vi "Retrieve Unit from Data Report.vi"(8 "error in (no error)":errorcluster, 10 "Row":u16, 11 "report in":refnum<class "NI_report.lvclass">) -> (0 "error out":errorcluster, 2 "data":string, 3 "report out":refnum<class "NI_report.lvclass">)   [LabVIEW 2019]
doc: "For use with Tektronix Excel Data Reports\n\nReturns the text in the Units column for the given Row (Zero Indexed)"
uses:
  <vilib>/Utility/NIReport.llb/NI_report.lvclass
  <vilib>/addons/_office/excel.llb/Excel Get Data (str).vi
  <vilib>/addons/_office/NI_ReportGenerationToolkit.lvlib
  <vilib>/Utility/NIReport.llb/Excel/NI_Excel.lvclass
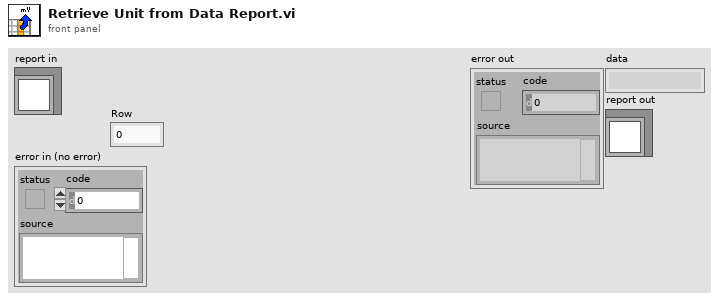
[diagram p1: front panel]
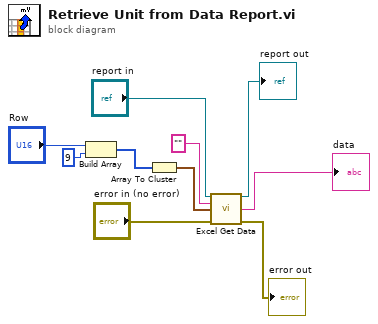
[diagram p0: block diagram]
diagram:
  n1 = Build Array("Row", u16 9 ("element")) -> (w9:u16[])
  n2 = Array To Cluster(array=w9) -> (cluster=w6:cluster{"[0]":u16, "[1]":u16})
  n3 = call-poly <vilib>:"Excel Get Data.vi"("report in"="report in", "data type"="", "start (0, 0)"=w6, "error in (no error)"="error in (no error)") -> ("report out"=→"report out":refnum<class "NI_report.lvclass">, "data"=→"data":string, "error out"=→"error out":errorcluster)  [unwired: 9 in]
